vi "svl_Autoscale.vi"(1 "scale":cluster{"min":dbl, "max":dbl} {"max" format="%.2f"; "min" format="%.2f"}) -> (0 "autoscale":cluster{"min":dbl, "max":dbl} {"max" format="%.2f"; "min" format="%.2f"})   [LabVIEW 2017]
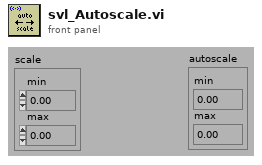
[diagram p1: front panel]
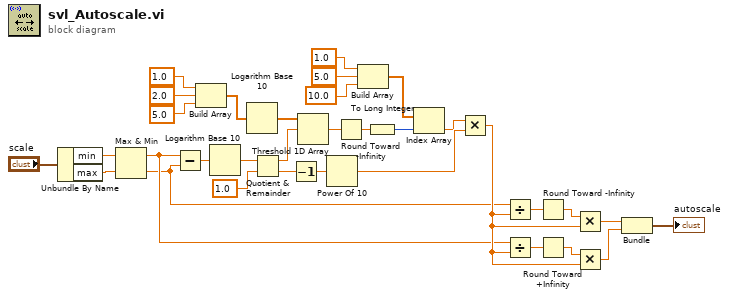
[diagram p0: block diagram]
diagram:
  n1 = Unbundle By Name("scale") -> ("min"=w2:dbl, "max"=w1:dbl)
  n2 = Max & Min(x=w2, y=w1) -> (max(x,y)=w4:dbl, min(x,y)=w3:dbl)
  n3 = Subtract(x=w4, y=w3) -> (x-y=w32:dbl)
  n4 = Build Array(1.0 ("x"), 2.0 ("x"), 5.0 ("x")) -> (w10:dbl[])
  n5 = Logarithm Base 10(1:w32) -> (0:w29:dbl)
  n6 = Logarithm Base 10(1:w10) -> (0:w26:dbl[])
  n7 = Quotient & Remainder(x=w29, y=1.0) -> (x-y*floor(x/y)=w25:dbl, floor(x/y)=w23:dbl)
  n8 = Decrement(x=w23) -> (x-1=w22:dbl)
  n9 = Threshold 1D Array(2:w25, 3:w26) -> (0:w21:dbl)  [unwired: 1 in]
  n10 = Power Of 10(x=w22) -> (10^x=w18:dbl)
  n11 = Round Toward -Infinity(1:w21) -> (0:w20:dbl)
  n12 = Build Array(1.0 ("x"), 5.0 ("x"), 10.0 ("x")) -> (w7:dbl[])
  n13 = To Long Integer(number=w20) -> (32bit integer=w19:i32)
  n14 = Index Array(array=w7, index=w19) -> (element=w17:dbl)
  n15 = Multiply(x=w17, y=w18) -> (x*y=w14:dbl)
  n16 = Divide(x=w3, y=w14) -> (x/y=w15:dbl)
  n17 = Divide(x=w4, y=w14) -> (x/y=w31:dbl)
  n18 = Round Toward -Infinity(1:w15) -> (0:w16:dbl)
  n19 = Round Toward +Infinity(x=w31) -> (ceil(x): smallest int >= x=w30:dbl)
  n20 = Multiply(x=w16, y=w14) -> (x*y=w13:dbl)
  n21 = Multiply(x=w30, y=w14) -> (x*y=w12:dbl)
  n22 = Bundle(w13, w12) -> (→"autoscale":cluster{dbl, dbl})  [unwired: 1 in]
